vi "Orifice Flow Calculator of Water In (((Pre))) Evaporation ASME.vi"(0 "Water Temperature":dbl[unit]=10.0 min=10.0 max=95.0, 1 "Delta P\n(Presure Made By Orifice)":dbl[unit], 2 "Orifice Diameter":dbl[unit]=0.01) -> (4 "Water Flow Pre Eva":bool, 5 "Mass Flow (Orifice) (Kg/min)":dbl[unit], 6 "Iteration Volumetric Flow \n(Orifice) (Lit/min)":dbl[unit])   [LabVIEW 2018]
panel:
  out "ReD":dbl
  out "Mass Flow (Orifice) (Kg/h)":dbl[unit](knob)
  out "Mass Flow (Orifice) (Kg/s)":dbl[unit]
  out "Pipe Velocity (m/s)":dbl[unit]
  out "Pipe Area (cm^2)":dbl[unit]
  out "Throat Velocity (m/s)":dbl[unit]
  out "Throat Area (cm^2)":dbl[unit]
  out "Beta":dbl
  out "orifice coefficient":dbl
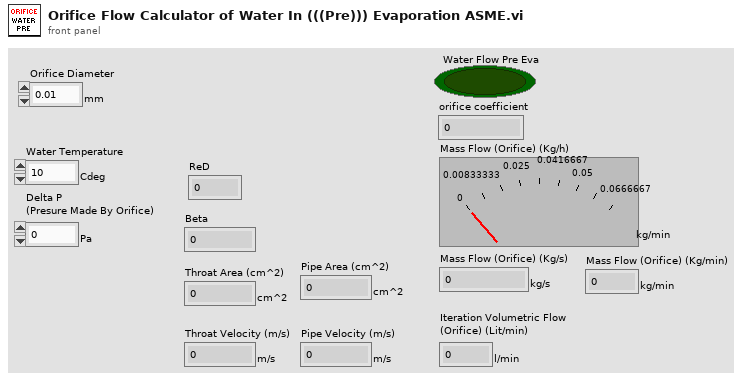
[diagram p1: front panel]
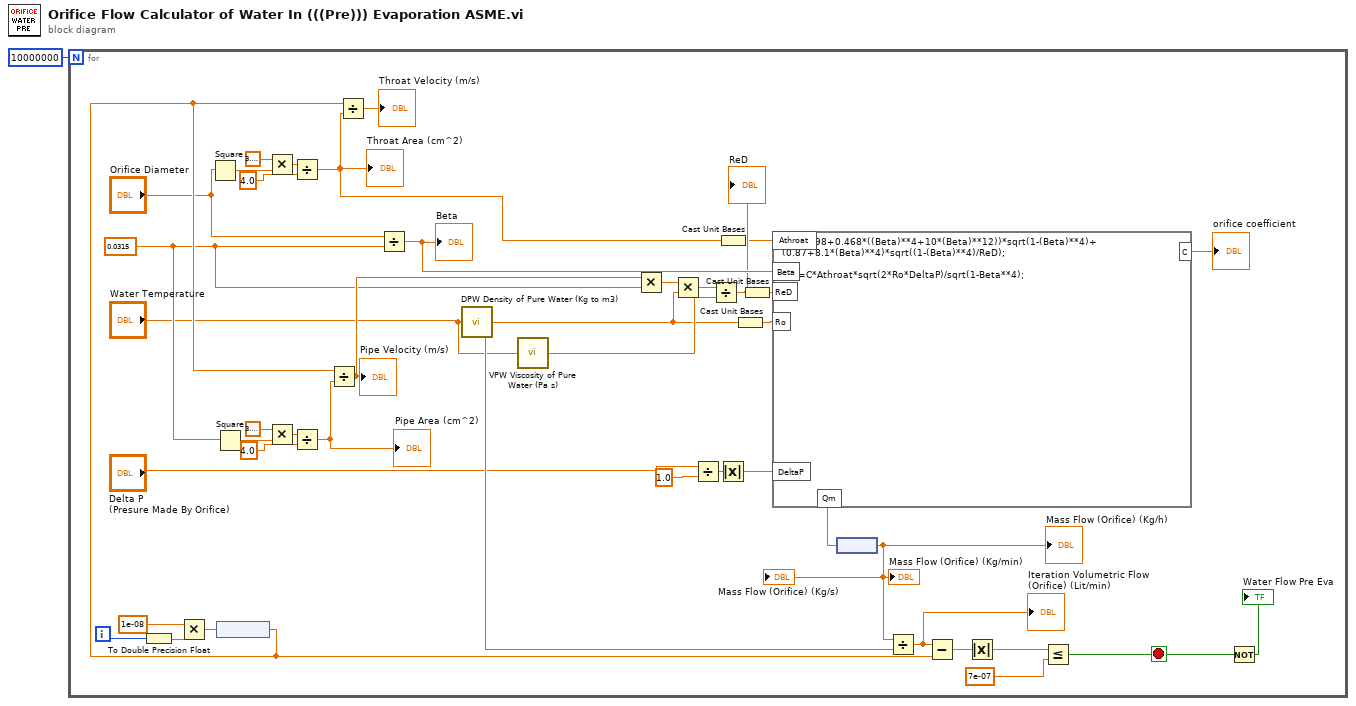
[diagram p0: block diagram]
diagram:
  n1 = for {
    N: 10000000 -> [_]
    i -> [w29]
    stop <- w5 stop-if-true
    w10 = dbl[unit] 0.0315 ("Pipe Diameter (mm)")
    n2 = To Double Precision Float(number=w29) -> (double precision float=w31:dbl)
    n3 = Multiply(x=1e-08, y=w31) -> (x*y=w4:dbl)
    n4 = Square(x="Orifice Diameter") -> (x^2=w40:dbl[unit])
    n5 = Square(x=w10) -> (x^2=w36:dbl[unit])
    n6 = node(w4) -> (w27:dbl[unit])
    n7 = Multiply(x=3.141592653589793, y=w40) -> (x*y=w42:dbl[unit])
    n8 = Multiply(x=3.141592653589793, y=w36) -> (x*y=w38:dbl[unit])
    n9 = Divide(x=w42, y=4.0) -> (x/y=w15:dbl[unit])
    "Throat Area (cm^2)" <- w15
    n10 = Divide(x=w38, y=4.0) -> (x/y=w35:dbl[unit])
    "Pipe Area (cm^2)" <- w35
    n11 = Divide(x=w27, y=w35) -> (x/y=w11:dbl[unit])
    "Pipe Velocity (m/s)" <- w11
    n12 = Divide(x=w27, y=w15) -> (x/y=→"Throat Velocity (m/s)":dbl[unit])
    n13 = Divide(x="Orifice Diameter", y=w10) -> (x/y=w23:dbl)
    "Beta" <- w23
    n14 = call "DPW Density of Pure Water (Kg to m3).vi"("Pure Water Temprature"="Water Temperature") -> ("DPW"=w12:dbl[unit])
    n15 = call "VPW Viscosity of Pure Water (Pa s).vi"("Pure Water Temprature"="Water Temperature") -> ("Visocity of pure Water (Pa S)"=w17:dbl[unit])
    n16 = Multiply(x=w11, y=w10) -> (x*y=w22:dbl[unit])
    n17 = Multiply(x=w22, y=w12) -> (x*y=w21:dbl[unit])
    n18 = Divide(x="Delta P\n(Presure Made By Orifice)", y=dbl[unit] 1.0) -> (x/y=w7:dbl)
    n19 = Divide(x=w21, y=w17) -> (x/y=w19:dbl)
    "ReD" <- w19
    n20 = Cast Unit Bases(0:w15) -> (2:w16:dbl)  [unwired: 1 in]
    n21 = Absolute Value(x=w7) -> (abs(x)=w3:dbl)
    n22 = Cast Unit Bases(0:w12) -> (2:w13:dbl)  [unwired: 1 in]
    n23 = Cast Unit Bases(0:w19) -> (2:w18:dbl)  [unwired: 1 in]
    n24 = formula code="C=(0.598+0.468*((Beta)**4+10*(Beta)**12))*sqrt(1-(Beta)**4)+\n(0.87+8.1*(Beta)**4)*sqrt((1-(Beta)**4)/ReD);\n\nQm=C*Athroat*sqrt(2*Ro*DeltaP)/sqrt(1-Beta**4);"("Beta"=w23, "Athroat"=w16, "Ro"=w13, "DeltaP"=w3, "ReD"=w18) -> ("C"=→"orifice coefficient":dbl, "Qm"=w34:dbl)
    n25 = node(w34) -> (w32:dbl[unit])
    "Mass Flow (Orifice) (Kg/s)" <- w32
    "Mass Flow (Orifice) (Kg/h)" <- w32
    "Mass Flow (Orifice) (Kg/min)" <- w32
    n26 = Divide(x=w32, y=w12) -> (x/y=w28:dbl[unit])
    "Iteration Volumetric Flow \n(Orifice) (Lit/min)" <- w28
    n27 = Subtract(x=w28, y=w27) -> (x-y=w26:dbl[unit])
    n28 = Absolute Value(x=w26) -> (abs(x)=w25:dbl[unit])
    n29 = Less Or Equal?(x=w25, y=dbl[unit] 7e-07) -> (x <= y?=w5:bool)
    n30 = Not(x=w5) -> (.not. x?=→"Water Flow Pre Eva":bool)
  }
